vi "Write Measurement Times.vi"(8 "error in (no error)":errorcluster, 10 "Measurement Times":string[](array[string]), 11 "SPECAN_PVT in":refnum<class "SPECAN_PVT.lvclass">) -> (0 "error out":errorcluster, 3 "SPECAN_PVT out":refnum<class "SPECAN_PVT.lvclass">)   [LabVIEW 2018, in "SPECAN_PVT.lvlib" / "SPECAN_PVT.lvclass"]
uses:
  SPECAN_PVT.lvclass
  SPECAN_PVT.lvclass/SPECAN_PVT.ctl
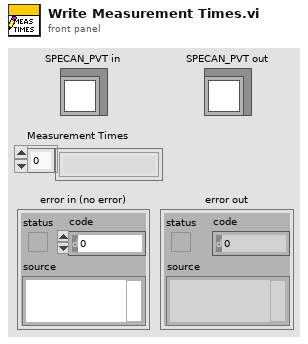
[diagram p1: front panel]
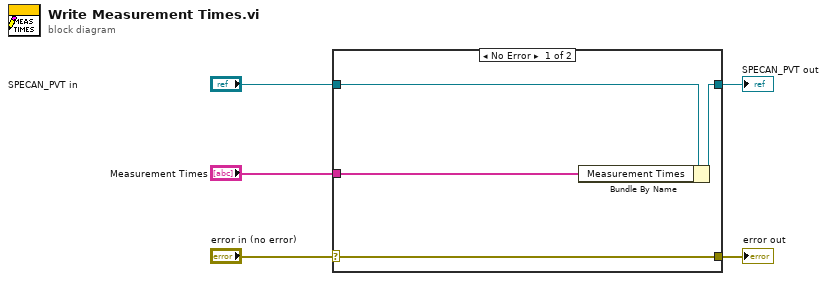
[diagram p0: block diagram]
diagram:
  n1 = case shown="No Error" "error in (no error)" {
    selector: "error in (no error)" -> [w9 w10]
    tunnel: [w9 w10] -> w4
    tunnel: [w7 w11] -> w2
    tunnel: "SPECAN_PVT in" -> [w8 w11]
    tunnel: "Measurement Times" -> [w6 _]
    frame No Error {
      n2 = Bundle By Name(cluster=w8, "Measurement Times"=w6) -> (w7:refnum<class "SPECAN_PVT.lvclass">)
    }
    frame Error {
    }
  }
  "error out" <- w4
  "SPECAN_PVT out" <- w2
